vi "MegaAnalysis5.vi"() -> ()   [LabVIEW 2016] (continued)
                    n131 = property on="data column selection" class="Arr (strict)"("Val(Sgnl)"=w337) -> ()  [unwired: 2 in, 2 out]
                  }
                }
              }
              frame #4 {
                n132 = case shown="False" "clear arrays" {
                  tunnel: w339 -> [_ w340]
                  frame False {
                  }
                  frame True {
                    n133 = property on="data column selection" class="Arr (strict)"("Val(Sgnl)"=w340) -> ()  [unwired: 2 in, 2 out]
                    n134 = property on="data column rescale" class="Arr (strict)"("Val(Sgnl)"=w340) -> ()  [unwired: 2 in, 2 out]
                    n135 = property on="data column offset" class="Arr (strict)"("Val(Sgnl)"=w340) -> ()  [unwired: 2 in, 2 out]
                  }
                }
              }
            }
          }
          frame #8 {
            n136 = case shown="True" "?" {
              frame False {
              }
              frame True {
                n137 = Build Array(path "") -> (w360:path[])
                n138 = property on="files to be imported" class="Arr (strict)"("Val(Sgnl)"=w360) -> ()  [unwired: 2 in, 2 out]
              }
            }
            n139 = case shown="False" "divide amplitude rescale amplitude by Sin(2 x angle of B field)" {
              tunnel: w341 -> [_ w358]
              tunnel: w343 -> [_ w359]
              frame False {
              }
              frame True {
                n140 = Unbundle(w359) -> ("data column rescale"=w349:ext[])  [unwired: 4 out]
                n141 = Divide(x=w358, y=180) -> (x/y=w356:ext[])
                n142 = Multiply(x=w356, y=3.141592653589793) -> (x*y=w354:ext[])
                n143 = Multiply(x=2, y=w354) -> (x*y=w352:ext[])
                n144 = Sine(x=w352) -> (sin(x)=w351:ext[])
                n145 = Divide(x=w349, y=w351) -> (x/y=w350:ext[])
                n146 = property on="data column rescale" class="Arr (strict)"("Val(Sgnl)"=w350) -> ()  [unwired: 2 in, 2 out]
              }
            }
            n147 = case shown="False" "increment all angles (theta) by:" {
              tunnel: w341 -> [_ w347]
              frame False {
              }
              frame True {
                n148 = Add(x="?", y=w347) -> (x+y=w346:ext[])
                n149 = property on="angle theta (cos theta renorm.)" class="Arr (strict)"("Val(Sgnl)"=w346) -> ()  [unwired: 2 in, 2 out]
              }
            }
          }
          frame #9 {
            n150 = for {
              tunnel: w374 -> [w379] mode=indexing
              tunnel: [w379] -> w373 mode=indexing
              tunnel: [w381] -> w364 mode=indexing
              tunnel: [w380] -> _ mode=indexing
              n151 = Strip Path(path=w379) -> (stripped path=w380:path, name=w381:string)
            }
            n152 = Build Array(w365, w364) -> (w362:string[][])
            n153 = Transpose 2D Array(2D array=w362) -> (transposed array=→"file list":string[][])
            n154 = case shown="True" w369 {
              tunnel: w378 -> [_ w391]
              tunnel: w377 -> [_ w395]
              tunnel: w376 -> [_ w394]
              tunnel: w375 -> [_ w393]
              tunnel: w373 -> [_ w390]
              tunnel: w372 -> [_ w389]
              tunnel: w371 -> [_ w388]
              tunnel: "file format" -> [_ w387]
              tunnel: w368 -> [_ w384]
              tunnel: w367 -> [_ w383]
              tunnel: w366 -> [_ w382]
              frame False {
              }
              frame True {
                n155 = for {
                  tunnel: w395 -> [w418]
                  tunnel: w391 -> [w417]
                  tunnel: w394 -> [w416]
                  tunnel: w393 -> [w415]
                  tunnel: w387 -> [w414]
                  tunnel: "skip" -> [w403]
                  tunnel: w390 -> [w399] mode=indexing
                  tunnel: w389 -> [w406]
                  tunnel: w388 -> [w405]
                  tunnel: [w404] -> w386 mode=indexing
                  tunnel: [w402] -> w385 mode=indexing
                  tunnel: w384 -> [w401]
                  tunnel: w383 -> [w397]
                  tunnel: w382 -> [w400]
                  i -> [w419]
                  n156 = call "tmdsverify.vi"("file path"=w399) -> ("Boolean"=w398:bool)  [unwired: 10 in]
                  n157 = case shown="True" w398 {
                    tunnel: w414 -> [w423 _]
                    tunnel: [w422 w426] -> w408
                    tunnel: w399 -> [w421 w427]
                    tunnel: w397 -> [w420 _]
                    tunnel: [w420 w425] -> w396
                    frame False {
                      n158 = call-poly <vilib>:"Read From Spreadsheet File.vi"("format (%.3f)"=w423, "file path (dialog if empty)"=w421) -> ("all rows"=w422:dbl[][])  [unwired: 2 in, 7 out]
                    }
                    frame True {
                      n159 = local read "Group name"() -> (w424:string)
                      n160 = call "TDMSextractspreadsheet.vi"("Group name"=w424, "file path"=w427) -> ("dt"=w425:dbl, "data"=w426:dbl[][])  [unwired: 7 in, 1 out]
                    }
                  }
                  n161 = Array Size(array=w408) -> (size(s)=w411:i32[])
                  n162 = Index Array(array=w411, index=0) -> (element=w410:i32)
                  n163 = Index Array(array=w411, index=1) -> (element=w402:i32)
                  n164 = Subtract(x=w410, y=w403) -> (x-y=w404:i32)
                  n165 = Array Subset(array=w408, index (row)=w403, length (row)=w404, index (col)=0, length (col)=w402) -> (w407:dbl[][])
                  n166 = stacked-sequence {
                    seq-local: [w434 _ _ _ _ _ _ _] -> [_ _ w531 w612 w680 _ _ _]
                    tunnel: w407 -> [w442 w483 w535 w613 w681 _ w756 _]
                    tunnel: w419 -> [w430 w474 w519 w599 w663 w731 w748 w758]
                    tunnel: w418 -> [w429 w473 w518 w598 w662 w730 w747 w759]
                    tunnel: w417 -> [w441 w484 w536 w614 w682 _ _ _]
                    tunnel: w416 -> [w440 w489 w539 w617 w685 _ _ _]
                    tunnel: w415 -> [w439 w490 w540 w618 w686 _ _ _]
                    tunnel: w406 -> [_ _ w530 w609 w679 _ _ _]
                    tunnel: w405 -> [_ _ w527 w602 w672 _ _ _]
                    tunnel: w401 -> [w432 w476 w521 w593 w661 w729 w751 w760]
                    tunnel: w396 -> [w428 _ _ _ _ _ _ _]
                    tunnel: w400 -> [_ _ w514 _ _ _ _ _]
                    frame #0 {
                      # "time"
                      n167 = Unbundle(w440) -> ("time column selection"=w438:u16[])  [unwired: 4 out]
                      n168 = Unbundle(w439) -> ("time column rescale"=w437:ext[])  [unwired: 4 out]
                      n169 = case shown="1" w441 {
                        tunnel: [w447 w450] -> w435
                        tunnel: [w446 w449] -> w436
                        tunnel: w438 -> [w445 w453]
                        tunnel: w437 -> [w444 w452]
                        tunnel: w430 -> [_ w451]
                        frame 0, Default {
                          w448 = 0
                          n170 = Index Array(array=w444, index=w448) -> (element=w446:ext)
                          n171 = Index Array(array=w445, index=w448) -> (element=w447:u16)
                        }
                        frame 1 {
                          n172 = Index Array(array=w453, index=w451) -> (element=w450:u16)
                          n173 = Index Array(array=w452, index=w451) -> (element=w449:ext)
                        }
                      }
                      n174 = case shown="2" "option" {
                        tunnel: [dbl[] [] ("Array 3") w457 w468] -> w433
                        tunnel: w442 -> [_ w465 w470]
                        tunnel: w436 -> [_ w463 _]
                        tunnel: w435 -> [_ w462 _]
                        tunnel: [w454 w456 w466] -> w434
                        tunnel: w428 -> [w454 _ w466]
                        frame 0, Default {
                        }
                        frame 1 {
                          n175 = Index Array(array=w465, index (col)=w462) -> (element=w464:dbl[])  [unwired: 1 in]
                          n176 = Multiply(x=w464, y=w463) -> (x*y=w457:ext[])
                          n177 = Index Array(array=w457, index=0) -> (element=w459:ext)
                          n178 = Index Array(array=w457, index=1) -> (element=w458:ext)
                          n179 = Subtract(x=w458, y=w459) -> (x-y=w456:ext)
                        }
                        frame 2 {
                          n180 = Index Array(array=w470, index (col)=0) -> (element=w469:dbl[])  [unwired: 1 in]
                          n181 = for {
                            tunnel: [w472] -> w467 mode=indexing
                            tunnel: w469 -> [_] mode=indexing
                            i -> [w472]
                          }
                          n182 = Multiply(x=w467, y=w466) -> (x*y=w468:dbl[])
                        }
                      }
                      n183 = property on="time interval  (for series)" class="DigNum (strict)"("Val(Sgnl)"=w428) -> ()  [unwired: 2 in, 2 out]
                      n184 = call "writebinary.vi"(7:w432, "base path"=w429, "file index"=w430, "data column"="time", "data"=w433) -> ()  [unwired: 7 out]
                    }
                    frame #1 {
                      w475 = "bdot"
                      (unwired) 3
                      # "bdot"
                      n185 = Unbundle(w489) -> ("dB/dt column selection"=w488:u16[])  [unwired: 4 out]
                      n186 = Unbundle(w490) -> ("dB/dt column rescale"=w487:ext[])  [unwired: 4 out]
                      n187 = case shown="1" w484 {
                        tunnel: [w495 w501] -> w486
                        tunnel: [w494 w500] -> w485
                        tunnel: w488 -> [w493 w499]
                        tunnel: w487 -> [w492 w498]
                        tunnel: w474 -> [_ w497]
                        frame 0, Default {
                          w496 = 0
                          n188 = Index Array(array=w492, index=w496) -> (element=w494:ext)
                          n189 = Index Array(array=w493, index=w496) -> (element=w495:u16)
                        }
                        frame 1 {
                          n190 = Index Array(array=w499, index=w497) -> (element=w501:u16)
                          n191 = Index Array(array=w498, index=w497) -> (element=w500:ext)
                        }
                      }
                      n192 = case shown="0, Default" "option" {
                        tunnel: [dbl[] [] ("Array 5") w505] -> w477
                        tunnel: w483 -> [_ w507]
                        tunnel: w486 -> [_ w504]
                        tunnel: w485 -> [_ w503]
                        frame 0, Default {
                        }
                        frame 1 {
                          n193 = Index Array(array=w507, index (col)=w504) -> (element=w506:dbl[])  [unwired: 1 in]
                          n194 = Multiply(x=w506, y=w503) -> (x*y=w505:ext[])
                        }
                      }
                      n195 = Number To Decimal String(number=w474, width (-)=2) -> (decimal integer string=w481:string)
                      n196 = call "writebinary.vi"(7:w476, "base path"=w473, "file index"=w474, "data column"=w475, "data"=w477) -> ()  [unwired: 7 out]
                      n197 = Search and Replace String(input string=w481, search string=" ", replace string="0") -> (result string=w478:string)  [unwired: 2 in, 6 out]
                      n198 = Concatenate Strings(w478, w475) -> ()  [unwired: 1 out]
                    }
                    frame #2 {
                      # "Bcol"
                      n199 = Unbundle(w539) -> ("B column selection"=w533:u16[])  [unwired: 4 out]
                      n200 = Unbundle(w540) -> ("B column rescale"=w532:ext[])  [unwired: 4 out]
                      n201 = Unbundle(w530) -> ("B column offset"=w529:ext[])  [unwired: 2 out]
                      n202 = case shown="1" w536 {
                        tunnel: [w562 w571] -> w538
                        tunnel: [w561 w570] -> w537
                        tunnel: w533 -> [w560 w569]
                        tunnel: w532 -> [w559 w568]
                        tunnel: w519 -> [_ w564]
                        tunnel: w529 -> [w558 w567]
                        tunnel: [w557 w566] -> w523
                        tunnel: w514 -> [w556 w563]
                        tunnel: [w555 w565] -> w512
                        frame 0, Default {
                          w554 = 0
                          n203 = Index Array(array=w558, index=w554) -> (element=w557:ext)
                          n204 = Index Array(array=w556, index=w554) -> (element=w555:ext)
                          n205 = Index Array(array=w559, index=w554) -> (element=w561:ext)
                          n206 = Index Array(array=w560, index=w554) -> (element=w562:u16)
                        }
                        frame 1 {
                          n207 = Index Array(array=w569, index=w564) -> (element=w571:u16)
                          n208 = Index Array(array=w567, index=w564) -> (element=w566:ext)
                          n209 = Index Array(array=w568, index=w564) -> (element=w570:ext)
                          n210 = Index Array(array=w563, index=w564) -> (element=w565:ext)
                        }
                      }
                      n211 = Unbundle(w527) -> ("pretrigger time for integration"=w526:dbl)  [unwired: 2 out]
                      n212 = case shown="0, Default" "option" {
                        tunnel: [dbl[] [] ("Array 6") w575 w582 w592] -> w525
                        tunnel: w535 -> [_ w577 w583 _]
                        tunnel: w538 -> [_ w574 w581 _]
                        tunnel: w537 -> [_ w573 w580 _]
                        tunnel: w531 -> [_ _ _ w591]
                        tunnel: w526 -> [_ _ _ w589]
                        tunnel: w521 -> [_ _ _ w588]
                        tunnel: w519 -> [_ _ _ w586]
                        tunnel: w518 -> [_ _ _ w585]
                        frame 0, Default {
                        }
                        frame 1 {
                          n213 = Index Array(array=w577, index (col)=w574) -> (element=w576:dbl[])  [unwired: 1 in]
                          n214 = Multiply(x=w576, y=w573) -> (x*y=w575:ext[])
                        }
                        frame 2 {
                          n215 = Index Array(array=w583, index (col)=w581) -> (element=w579:dbl[])  [unwired: 1 in]
                          n216 = Reciprocal(x=w579) -> (1/x=w578:dbl[])
                          n217 = Multiply(x=w578, y=w580) -> (x*y=w582:ext[])
                        }
                        frame 3 {
                          n218 = call "readbinary.vi"(7:w588, "base path"=w585, "file index"=w586, "data column"="bdot") -> ("data"=w584:ext[])  [unwired: 7 out]
                          n219 = call "integrator2.vi"("reverse intergral"="?", "pretrigger t"=w589, "dt"=w591, "data"=w584) -> ("integrated data"=w592:dbl[])  [unwired: 2 in]
                        }
                      }
                      n220 = Divide(x=w512, y=180) -> (x/y=w516:ext)
                      n221 = Multiply(x=w516, y=3.141592653589793) -> (x*y=w513:ext)
                      n222 = Cosine(x=w513) -> (cos(x)=w511:ext)
                      n223 = case shown="True" "?" {
                        tunnel: w525 -> [w544 w546]
                        tunnel: [w544 w545] -> w524
                        frame False {
                        }
                        frame True {
                          n224 = Absolute Value(x=w546) -> (abs(x)=w550:ext[])
                          n225 = Array Max & Min(array=w550) -> (max index (indices)=w549:i32)  [unwired: 3 out]
                          n226 = Index Array(array=w546, index=w549) -> (element=w548:ext)
                          n227 = Sign(1:w548) -> (0:w547:ext)
                          n228 = Multiply(x=w546, y=w547) -> (x*y=w545:ext[])
                        }
                      }
                      n229 = case shown="False" "?" {
                        tunnel: w523 -> [w542 w543]
                        tunnel: [w541 w543] -> _
                        frame False {
                          n230 = To Double Precision Float(number=w542) -> (double precision float=w541:dbl)
                        }
                        frame True {
                        }
                      }
                      n231 = case shown="False" "?" {
                        tunnel: w524 -> [w551 w553]
                        tunnel: [w551 w552] -> w510
                        frame False {
                        }
                        frame True {
                          n232 = call "forceBendtozero2.vi"("data"=w553) -> ("forced data"=w552:dbl[])
                        }
                      }
                      n233 = Add(x=w523, y=w510) -> (x+y=w509:ext[])
                      n234 = Multiply(x=w509, y=w511) -> (x*y=w508:ext[])
                      n235 = call "writebinary.vi"(7:w521, "base path"=w518, "file index"=w519, "data column"="bcol", "data"=w508) -> ()  [unwired: 7 out]
                    }
                    frame #3 {
                      # "data1"
                      n236 = Unbundle(w617) -> ("data column selection"=w610:u16[])  [unwired: 4 out]
                      n237 = Unbundle(w618) -> ("data column rescale"=w611:ext[])  [unwired: 4 out]
                      n238 = Unbundle(w609) -> ("data column offset"=w608:ext[])  [unwired: 2 out]
                      n239 = case shown="0, Default" w614 {
                        tunnel: [w632 w639] -> w616
                        tunnel: [w631 w638] -> w615
                        tunnel: w610 -> [w630 w637]
                        tunnel: w611 -> [w629 w636]
                        tunnel: w599 -> [_ w634]
                        tunnel: w608 -> [w628 w635]
                        tunnel: [w626 w633] -> w607
                        frame 0, Default {
                          w627 = 0
                          n240 = Index Array(array=w628, index=w627) -> (element=w626:ext)
                          n241 = Index Array(array=w629, index=w627) -> (element=w631:ext)
                          n242 = Index Array(array=w630, index=w627) -> (element=w632:u16)
                        }
                        frame 1 {
                          n243 = Index Array(array=w635, index=w634) -> (element=w633:ext)
                          n244 = Index Array(array=w637, index=w634) -> (element=w639:u16)
                          n245 = Index Array(array=w636, index=w634) -> (element=w638:ext)
                        }
                      }
                      n246 = Unbundle(w602) -> ("pretrigger time for integration"=w601:dbl)  [unwired: 2 out]
                      n247 = case shown="0, Default" "option" {
                        tunnel: [dbl[] [] ("Array 7") w643 w650 w660] -> w604
                        tunnel: w613 -> [_ w645 w651 w657]
                        tunnel: w616 -> [_ w642 w649 w656]
                        tunnel: w615 -> [_ w641 w648 w652]
                        tunnel: w612 -> [_ _ _ w659]
                        tunnel: w601 -> [_ _ _ w654]
                        frame 0, Default {
                        }
                        frame 1 {
                          n248 = Index Array(array=w645, index (col)=w642) -> (element=w644:dbl[])  [unwired: 1 in]
                          n249 = Multiply(x=w644, y=w641) -> (x*y=w643:ext[])
                        }
                        frame 2 {
                          n250 = Index Array(array=w651, index (col)=w649) -> (element=w647:dbl[])  [unwired: 1 in]
                          n251 = Reciprocal(x=w647) -> (1/x=w646:dbl[])
                          n252 = Multiply(x=w646, y=w648) -> (x*y=w650:ext[])
                        }
                        frame 3 {
                          n253 = Index Array(array=w657, index (col)=w656) -> (element=w655:dbl[])  [unwired: 1 in]
                          n254 = Multiply(x=w652, y=w655) -> (x*y=w653:ext[])
                          n255 = call "integrator2.vi"("reverse intergral"="?", "pretrigger t"=w654, "dt"=w659, "data"=w653) -> ("integrated data"=w660:dbl[])  [unwired: 2 in]
                        }
                      }
                      n256 = case shown="False" "?" {
                        tunnel: w604 -> [w623 w625]
                        tunnel: [w623 w624] -> w603
                        frame False {
                        }
                        frame True {
                          n257 = call "forceBendtozero2.vi"("data"=w625) -> ("forced data"=w624:dbl[])
                        }
                      }
                      n258 = Add(x=w607, y=w603) -> (x+y=w596:ext[])
                      n259 = case shown="True" "?" {
                        tunnel: w596 -> [w619 w622]
                        tunnel: "?" -> [_ w621]
                        tunnel: [w619 w620] -> w594
                        frame False {
                        }
                        frame True {
                          n260 = Rotate 1D Array(1:w622, 2:w621) -> (0:w620:ext[])
                        }
                      }
                      n261 = call "writebinary.vi"(7:w593, "base path"=w598, "file index"=w599, "data column"="dat1", "data"=w594) -> ()  [unwired: 7 out]
                    }
                    frame #4 {
                      # "data2"
                      n262 = Unbundle(w685) -> ("data column selection"=w669:u16[])  [unwired: 4 out]
                      n263 = Unbundle(w686) -> ("data column rescale"=w670:ext[])  [unwired: 4 out]
                      n264 = Unbundle(w679) -> ("data column offset"=w678:ext[])  [unwired: 2 out]
                      n265 = case shown="0, Default" w682 {
                        tunnel: [w700 w707] -> w684
                        tunnel: [w699 w706] -> w683
                        tunnel: w669 -> [w698 w705]
                        tunnel: w670 -> [w697 w704]
                        tunnel: w663 -> [_ w702]
                        tunnel: w678 -> [w696 w703]
                        tunnel: [w694 w701] -> w677
                        frame 0, Default {
                          w695 = 0
                          n266 = Index Array(array=w696, index=w695) -> (element=w694:ext)
                          n267 = Index Array(array=w697, index=w695) -> (element=w699:ext)
                          n268 = Index Array(array=w698, index=w695) -> (element=w700:u16)
                        }
                        frame 1 {
                          n269 = Index Array(array=w703, index=w702) -> (element=w701:ext)
                          n270 = Index Array(array=w705, index=w702) -> (element=w707:u16)
                          n271 = Index Array(array=w704, index=w702) -> (element=w706:ext)
                        }
                      }
                      n272 = Unbundle(w672) -> ("pretrigger time for integration"=w671:dbl)  [unwired: 2 out]
                      n273 = case shown="0, Default" "option" {
                        tunnel: [dbl[] [] ("Array 8") w711 w718 w728] -> w673
                        tunnel: w681 -> [_ w713 w719 w726]
                        tunnel: w684 -> [_ w710 w717 w725]
                        tunnel: w683 -> [_ w709 w716 w720]
                        tunnel: w680 -> [_ _ _ w727]
                        tunnel: w671 -> [_ _ _ w722]
                        frame 0, Default {
                        }
                        frame 1 {
                          n274 = Index Array(array=w713, index (col)=w710) -> (element=w712:dbl[])  [unwired: 1 in]
                          n275 = Multiply(x=w712, y=w709) -> (x*y=w711:ext[])
                        }
                        frame 2 {
                          n276 = Index Array(array=w719, index (col)=w717) -> (element=w715:dbl[])  [unwired: 1 in]
                          n277 = Reciprocal(x=w715) -> (1/x=w714:dbl[])
                          n278 = Multiply(x=w714, y=w716) -> (x*y=w718:ext[])
                        }
                        frame 3 {
                          n279 = Index Array(array=w726, index (col)=w725) -> (element=w724:dbl[])  [unwired: 1 in]
                          n280 = Multiply(x=w720, y=w724) -> (x*y=w721:ext[])
                          n281 = call "integrator2.vi"("reverse intergral"="?", "pretrigger t"=w722, "dt"=w727, "data"=w721) -> ("integrated data"=w728:dbl[])  [unwired: 2 in]
                        }
                      }
                      n282 = case shown="False" "?" {
                        tunnel: w673 -> [w691 w693]
                        tunnel: [w691 w692] -> w674
                        frame False {
                        }
                        frame True {
                          n283 = call "forceBendtozero2.vi"("data"=w693) -> ("forced data"=w692:dbl[])
                        }
                      }
                      n284 = Add(x=w677, y=w674) -> (x+y=w668:ext[])
                      n285 = case shown="True" "?" {
                        tunnel: w668 -> [w687 w690]
                        tunnel: "?" -> [_ w689]
                        tunnel: [w687 w688] -> w665
                        frame False {
                        }
                        frame True {
                          n286 = Rotate 1D Array(1:w690, 2:w689) -> (0:w688:ext[])
                        }
                      }
                      n287 = call "writebinary.vi"(7:w661, "base path"=w662, "file index"=w663, "data column"="dat2", "data"=w665) -> ()  [unwired: 7 out]
                    }
                    frame #5 {
                      n288 = case shown="True" "?" {
                        tunnel: w731 -> [_ w735]
                        tunnel: w730 -> [_ w733]
                        tunnel: w729 -> [_ w734]
                        frame False {
                        }
                        frame True {
                          w742 = -1
                          n289 = call "readbinary.vi"(7:w734, "base path"=w733, "file index"=w735, "data column"="time") -> ("data"=w740:ext[])  [unwired: 7 out]
                          n290 = call "readbinary.vi"(7:w734, "base path"=w733, "file index"=w735, "data column"="bcol") -> ("data"=w743:ext[])  [unwired: 7 out]
                          n291 = Rotate 1D Array(1:w740, 2:w742) -> (0:w741:ext[])
                          n292 = Rotate 1D Array(1:w743, 2:w742) -> (0:w744:ext[])
                          n293 = Subtract(x=w740, y=w741) -> (x-y=w738:ext[])
                          n294 = Subtract(x=w743, y=w744) -> (x-y=w739:ext[])
                          n295 = Divide(x=w739, y=w738) -> (x/y=w737:ext[])
                          n296 = call "writebinary.vi"(7:w734, "base path"=w733, "file index"=w735, "data column"="bdot", "data"=w737) -> ()  [unwired: 7 out]
                        }
                      }
                    }
                    frame #6 {
                      n297 = Array Size(array=w756) -> (size(s)=w755:i32[])
                      n298 = Index Array(array=w755, index=0) -> (element=w753:i32)
                      n299 = for {
                        N: w753 -> [_]
                        tunnel: [w757] -> w752 mode=indexing
                        i -> [w757]
                      }
                      n300 = To Extended Precision Float(1:w752) -> (0:w750:ext[])
                      n301 = call "writebinary.vi"(7:w751, "base path"=w747, "file index"=w748, "data column"="indx", "data"=w750) -> ()  [unwired: 7 out]
                    }
                    frame #7 {
                      n302 = case shown="True" "?" {
                        tunnel: w760 -> [_ w764]
                        tunnel: w759 -> [_ w765]
                        tunnel: w758 -> [_ w766]
                        frame False {
                        }
                        frame True {
                          w784 = dbl[] [] ("Array 25")
                          n303 = call "readbinary.vi"(7:w764, "base path"=w765, "file index"=w766, "data column"="dat2") -> ("data"=w783:ext[])  [unwired: 7 out]
                          n304 = call "readbinary.vi"(7:w764, "base path"=w765, "file index"=w766, "data column"="indx") -> ("data"=w763:ext[])  [unwired: 7 out]
                          n305 = Array Size(array=w763) -> (size(s)=w762:i32)
                          n306 = call "readbinary.vi"(7:w764, "base path"=w765, "file index"=w766, "data column"="dat1") -> ("data"=w782:ext[])  [unwired: 7 out]
                          n307 = call "readbinary.vi"(7:w764, "base path"=w765, "file index"=w766, "data column"="time") -> ("data"=w780:ext[])  [unwired: 7 out]
                          n308 = call "readbinary.vi"(7:w764, "base path"=w765, "file index"=w766, "data column"="bdot") -> ("data"=w781:ext[])  [unwired: 7 out]
                          n309 = call "readbinary.vi"(7:w764, "base path"=w765, "file index"=w766, "data column"="bcol") -> ("data"=w779:ext[])  [unwired: 7 out]
                          n310 = for {
                            N: w762 -> [_]
                            shift-right: [w807] -> w778
                            shift-left: w784 -> [w808]
                            shift-right: [w805] -> w777
                            shift-left: w784 -> [w806]
                            shift-right: [w804] -> w776
                            shift-left: w784 -> [w803]
                            shift-right: [w802] -> w775
                            shift-left: w784 -> [w801]
                            shift-right: [w800] -> w774
                            shift-left: w784 -> [w799]
                            shift-right: [w798] -> w773
                            shift-left: w784 -> [w797]
                            tunnel: w763 -> [w816]
                            tunnel: w783 -> [w815]
                            tunnel: w782 -> [w814]
                            tunnel: w781 -> [w813]
                            tunnel: w780 -> [w812]
                            tunnel: w779 -> [w811]
                            i -> [w810]
                            n311 = Index Array(array=w812, index=w810) -> (element=w795:ext)
                            n312 = Index Array(array=w816, index=w810) -> (element=w791:ext)
                            n313 = Index Array(array=w815, index=w810) -> (element=w792:ext)
                            n314 = Index Array(array=w811, index=w810) -> (element=w796:ext)
                            n315 = Equal To 0?(x=w796) -> (x = 0?=w809:bool)
                            n316 = Index Array(array=w814, index=w810) -> (element=w793:ext)
                            n317 = Index Array(array=w813, index=w810) -> (element=w794:ext)
                            n318 = case shown="False" w809 {
                              tunnel: w808 -> [w834 w840]
                              tunnel: [w822 w840] -> w807
                              tunnel: w806 -> [w833 w839]
                              tunnel: [w821 w839] -> w805
                              tunnel: [w818 w838] -> w804
                              tunnel: w803 -> [w832 w838]
                              tunnel: [w819 w837] -> w802
                              tunnel: w801 -> [w831 w837]
                              tunnel: [w820 w836] -> w800
                              tunnel: w799 -> [w830 w836]
                              tunnel: [w817 w835] -> w798
                              tunnel: w797 -> [w829 w835]
                              tunnel: w796 -> [w828 _]
                              tunnel: w795 -> [w827 _]
                              tunnel: w794 -> [w826 _]
                              tunnel: w793 -> [w825 _]
                              tunnel: w792 -> [w824 _]
                              tunnel: w791 -> [w823 _]
                              frame False {
                                n319 = Build Array (concatenate)(w829, w823) -> (w817:ext[])
                                n320 = Build Array (concatenate)(w830, w824) -> (w820:ext[])
                                n321 = Build Array (concatenate)(w833, w827) -> (w821:ext[])
                                n322 = Build Array (concatenate)(w831, w825) -> (w819:ext[])
                                n323 = Build Array (concatenate)(w834, w828) -> (w822:ext[])
                                n324 = Build Array (concatenate)(w832, w826) -> (w818:ext[])
                              }
                              frame True {
                              }
                            }
                          }
                          n325 = call "writebinary.vi"(7:w764, "base path"=w765, "file index"=w766, "data column"="dat2", "data"=w774) -> ()  [unwired: 7 out]
                          n326 = call "writebinary.vi"(7:w764, "base path"=w765, "file index"=w766, "data column"="time", "data"=w777) -> ()  [unwired: 7 out]
                          n327 = call "writebinary.vi"(7:w764, "base path"=w765, "file index"=w766, "data column"="indx", "data"=w773) -> ()  [unwired: 7 out]
                          n328 = call "writebinary.vi"(7:w764, "base path"=w765, "file index"=w766, "data column"="dat1", "data"=w775) -> ()  [unwired: 7 out]
                          n329 = call "writebinary.vi"(7:w764, "base path"=w765, "file index"=w766, "data column"="bcol", "data"=w778) -> ()  [unwired: 7 out]
                          n330 = call "writebinary.vi"(7:w764, "base path"=w765, "file index"=w766, "data column"="bdot", "data"=w776) -> ()  [unwired: 7 out]
                        }
                      }
                    }
                  }
                }
                "# columns" <- w385
                "# rows" <- w386
              }
            }
          }
          frame #10 {
            n331 = case shown="True" "read angle from data 2 index:" {
              tunnel: w844 -> [_ w848]
              tunnel: w843 -> [_ w849]
              tunnel: w842 -> [_ w847]
              frame False {
              }
              frame True {
                n332 = for {
                  tunnel: w849 -> [w856]
                  tunnel: w848 -> [_] mode=indexing
                  tunnel: w847 -> [w854]
                  tunnel: "?" -> [w852]
                  tunnel: [w850] -> w845 mode=indexing
                  i -> [w853]
                  n333 = call "readbinary.vi"(7:w856, "base path"=w854, "file index"=w853, "data column"="dat2") -> ("data"=w851:ext[])  [unwired: 7 out]
                  n334 = Index Array(array=w851, index=w852) -> (element=w850:ext)
                }
                n335 = property on="angle theta (cos theta renorm.)" class="Arr (strict)"("Val(Sgnl)"=w845) -> ()  [unwired: 2 in, 2 out]
              }
            }
          }
          frame #11 {
            n336 = case shown="True" "make all files have same settings as file 0" {
              tunnel: w857 -> [_ w859]
              frame False {
              }
              frame True {
                n337 = stacked-sequence {
                  tunnel: w859 -> [w860 w871 w891 w906 w925]
                  frame #0 {
                    n338 = property on="time column selection" class="Arr (strict)"() -> ("Value"=w864:u16[])  [unwired: 2 in, 2 out]
                    n339 = property on="time column rescale" class="Arr (strict)"() -> ("Value"=w863:ext[])  [unwired: 2 in, 2 out]
                    n340 = Index Array(array=w864, index=0) -> (element=w866:u16)
                    n341 = Index Array(array=w863, index=0) -> (element=w865:ext)
                    n342 = for {
                      tunnel: w866 -> [w870]
                      tunnel: w865 -> [w869]
                      tunnel: [w870] -> w862 mode=indexing
                      tunnel: [w869] -> w861 mode=indexing
                      tunnel: w860 -> [_] mode=indexing
                    }
                    n343 = property on="time column selection" class="Arr (strict)"("Val(Sgnl)"=w862) -> ()  [unwired: 2 in, 2 out]
                    n344 = property on="time column rescale" class="Arr (strict)"("Val(Sgnl)"=w861) -> ()  [unwired: 2 in, 2 out]
                  }
                  frame #1 {
                    n345 = property on="dB/dt column rescale" class="Arr (strict)"() -> ("Value"=w874:ext[])  [unwired: 2 in, 2 out]
                    n346 = property on="dB/dt column selection" class="Arr (strict)"() -> ("Value"=w875:u16[])  [unwired: 2 in, 2 out]
                    n347 = Index Array(array=w875, index=0) -> (element=w877:u16)
                    n348 = Index Array(array=w874, index=0) -> (element=w876:ext)
                    n349 = for {
                      tunnel: w877 -> [w881]
                      tunnel: w876 -> [w880]
                      tunnel: [w881] -> w873 mode=indexing
                      tunnel: [w880] -> w872 mode=indexing
                      tunnel: w871 -> [_] mode=indexing
                    }
                    n350 = property on="dB/dt column rescale" class="Arr (strict)"("Val(Sgnl)"=w872) -> ()  [unwired: 2 in, 2 out]
                    n351 = property on="dB/dt column selection" class="Arr (strict)"("Val(Sgnl)"=w873) -> ()  [unwired: 2 in, 2 out]
                  }
                  frame #2 {
                    n352 = local read "B column selection"() -> (w882:u16[])
                    n353 = property on="B column rescale" class="Arr (strict)"() -> ("Value"=w894:ext[])  [unwired: 2 in, 2 out]
                    n354 = property on="angle theta (cos theta renorm.)" class="Arr (strict)"() -> ("Value"=w893:ext[])  [unwired: 2 in, 2 out]
                    n355 = property on="B column offset" class="Arr (strict)"() -> ("Value"=w892:ext[])  [unwired: 2 in, 2 out]
                    n356 = Index Array(array=w882, index=0) -> (element=w890:u16)
                    n357 = Index Array(array=w892, index=0) -> (element=w887:ext)
                    n358 = Index Array(array=w894, index=0) -> (element=w889:ext)
                    n359 = Index Array(array=w893, index=0) -> (element=w888:ext)
                    n360 = for {
                      tunnel: w891 -> [_] mode=indexing
                      tunnel: w890 -> [w902]
                      tunnel: w889 -> [w901]
                      tunnel: w888 -> [w900]
                      tunnel: w887 -> [w899]
                      tunnel: [w902] -> w883 mode=indexing
                      tunnel: [w901] -> w886 mode=indexing
                      tunnel: [w900] -> w885 mode=indexing
                      tunnel: [w899] -> w884 mode=indexing
                    }
                    n361 = property on="B column offset" class="Arr (strict)"("Val(Sgnl)"=w884) -> ()  [unwired: 2 in, 2 out]
                    n362 = property on="angle theta (cos theta renorm.)" class="Arr (strict)"("Val(Sgnl)"=w885) -> ()  [unwired: 2 in, 2 out]
                    n363 = property on="B column rescale" class="Arr (strict)"("Val(Sgnl)"=w886) -> ()  [unwired: 2 in, 2 out]
                    n364 = local write "B column selection"(w883) -> ()
                  }
                  frame #3 {
                    n365 = property on="data column rescale" class="Arr (strict)"() -> ("Value"=w908:ext[])  [unwired: 2 in, 2 out]
                    n366 = property on="data column selection" class="Arr (strict)"() -> ("Value"=w909:u16[])  [unwired: 2 in, 2 out]
                    n367 = property on="data column offset" class="Arr (strict)"() -> ("Value"=w907:ext[])  [unwired: 2 in, 2 out]
                    n368 = Index Array(array=w909, index=0) -> (element=w912:u16)
                    n369 = Index Array(array=w908, index=0) -> (element=w911:ext)
                    n370 = Index Array(array=w907, index=0) -> (element=w910:ext)
                    n371 = for {
                      tunnel: w912 -> [w918]
                      tunnel: w911 -> [w917]
                      tunnel: w910 -> [w916]
                      tunnel: [w918] -> w905 mode=indexing
                      tunnel: [w917] -> w904 mode=indexing
                      tunnel: [w916] -> w903 mode=indexing
                      tunnel: w906 -> [_] mode=indexing
                    }
                    n372 = property on="data column rescale" class="Arr (strict)"("Val(Sgnl)"=w904) -> ()  [unwired: 2 in, 2 out]
                    n373 = property on="data column offset" class="Arr (strict)"("Val(Sgnl)"=w903) -> ()  [unwired: 2 in, 2 out]
                    n374 = property on="data column selection" class="Arr (strict)"("Val(Sgnl)"=w905) -> ()  [unwired: 2 in, 2 out]
                  }
                  frame #4 {
                    n375 = property on="data column rescale" class="Arr (strict)"() -> ("Value"=w923:ext[])  [unwired: 2 in, 2 out]
                    n376 = property on="data column selection" class="Arr (strict)"() -> ("Value"=w924:u16[])  [unwired: 2 in, 2 out]
                    n377 = property on="data column offset" class="Arr (strict)"() -> ("Value"=w922:ext[])  [unwired: 2 in, 2 out]
                    n378 = Index Array(array=w924, index=0) -> (element=w928:u16)
                    n379 = Index Array(array=w923, index=0) -> (element=w927:ext)
                    n380 = Index Array(array=w922, index=0) -> (element=w926:ext)
                    n381 = for {
                      tunnel: w928 -> [w934]
                      tunnel: w927 -> [w933]
                      tunnel: w926 -> [w932]
                      tunnel: [w934] -> w921 mode=indexing
                      tunnel: [w933] -> w920 mode=indexing
                      tunnel: [w932] -> w919 mode=indexing
                      tunnel: w925 -> [_] mode=indexing
                    }
                    n382 = property on="data column rescale" class="Arr (strict)"("Val(Sgnl)"=w920) -> ()  [unwired: 2 in, 2 out]
                    n383 = property on="data column selection" class="Arr (strict)"("Val(Sgnl)"=w921) -> ()  [unwired: 2 in, 2 out]
                    n384 = property on="data column offset" class="Arr (strict)"("Val(Sgnl)"=w919) -> ()  [unwired: 2 in, 2 out]
                  }
                }
              }
            }
          }
          frame #12 {
            n385 = case shown="0, Default" "sampling frequency option" {
              tunnel: w940 -> [w944 w957]
              tunnel: w939 -> [w943 _]
              tunnel: [w942 w955] -> w938
              tunnel: w937 -> [w941 _]
              tunnel: w935 -> [_ w956]
              frame 0, Default {
                n386 = for {
                  tunnel: w944 -> [_] mode=indexing
                  tunnel: w943 -> [w952]
                  tunnel: [w946] -> w942 mode=indexing
                  tunnel: w941 -> [w945]
                  i -> [w953]
                  n387 = call "readbinary.vi"(7:w945, "base path"=w952, "file index"=w953, "data column"="time") -> ("data"=w947:ext[])  [unwired: 7 out]
                  n388 = Index Array(array=w947, index=1) -> (element=w950:ext)
                  n389 = Index Array(array=w947, index=0) -> (element=w951:ext)
                  n390 = Subtract(x=w950, y=w951) -> (x-y=w946:ext)
                }
              }
              frame 1 {
                n391 = for {
                  tunnel: w957 -> [_] mode=indexing
                  tunnel: w956 -> [w958]
                  tunnel: [w958] -> w955 mode=indexing
                }
              }
            }
          }
          frame #13 {
            n392 = And(x="?", y=w960) -> (x .and. y?=w961:bool)
            n393 = case shown="True" w961 {
              tunnel: w965 -> [_ w969]
              tunnel: w964 -> [_ w968]
              tunnel: w963 -> [_ w967]
              tunnel: w959 -> [_ w966]
              frame False {
              }
              frame True {
                n394 = for {
                  tunnel: w969 -> [_] mode=indexing
                  tunnel: w968 -> [w973]
                  tunnel: w967 -> [w972]
                  tunnel: w966 -> [w970]
                  i -> [w971]
                  n395 = for {
                    tunnel: w973 -> [w977] mode=indexing
                    tunnel: w972 -> [w976]
                    tunnel: w971 -> [w975]
                    tunnel: w970 -> [w974]
                    n396 = call "readbinary.vi"(7:w974, "base path"=w976, "file index"=w975, "data column"=w977) -> ("data"=w981:ext[])  [unwired: 7 out]
                    n397 = Subtract(x="upper cutoff", y="lower cutoff") -> (x-y=w982:u64)
                    n398 = Increment(x=w982) -> (x+1=w979:u64)
                    n399 = Array Subset(array=w981, index="lower cutoff", length=w979) -> (w978:ext[])
                    n400 = call "writebinary.vi"(7:w974, "base path"=w976, "file index"=w975, "data column"=w977, "data"=w978) -> ()  [unwired: 7 out]
                  }
                }
              }
            }
          }
          frame #14 {
            n401 = And(x="?", y=w986) -> (x .and. y?=w985:bool)
            n402 = case shown="False" w985 {
              tunnel: w990 -> [_ w994]
              tunnel: w989 -> [_ w993]
              tunnel: w988 -> [_ w992]
              tunnel: w984 -> [_ w991]
              frame False {
              }
              frame True {
                n403 = for {
                  tunnel: w994 -> [w997]
                  tunnel: w992 -> [w996]
                  tunnel: w993 -> [_] mode=indexing
                  tunnel: w991 -> [w995]
                  i -> [w998]
                  n404 = stacked-sequence {
                    seq-local: [w1006 _] -> [_ w1014]
                    seq-local: [w1002 _] -> [_ w1013]
                    tunnel: w998 -> [w1010 w1016]
                    tunnel: w997 -> [w1009 w1015]
                    tunnel: w996 -> [_ w1017]
                    tunnel: w995 -> [w999 w1012]
                    frame #0 {
                      n405 = call "readbinary.vi"(7:w999, "base path"=w1009, "file index"=w1010, "data column"="time") -> ("data"=w1003:ext[])  [unwired: 7 out]
                      n406 = Subtract(x=w1003, y="lower cutoff") -> (x-y=w1008:ext[])
                      n407 = Subtract(x=w1003, y="upper cutoff") -> (x-y=w1005:ext[])
                      n408 = Absolute Value(x=w1008) -> (abs(x)=w1007:ext[])
                      n409 = Absolute Value(x=w1005) -> (abs(x)=w1004:ext[])
                      n410 = Array Max & Min(array=w1007) -> (min index (indices)=w1006:i32)  [unwired: 3 out]
                      n411 = Array Max & Min(array=w1004) -> (min index (indices)=w1002:i32)  [unwired: 3 out]
                    }
                    frame #1 {
                      n412 = for {
                        tunnel: w1017 -> [w1023] mode=indexing
                        tunnel: w1016 -> [w1022]
                        tunnel: w1015 -> [w1021]
                        tunnel: w1014 -> [w1019]
                        tunnel: w1013 -> [w1020]
                        tunnel: w1012 -> [w1018]
                        n413 = call "readbinary.vi"(7:w1018, "base path"=w1021, "file index"=w1022, "data column"=w1023) -> ("data"=w1026:ext[])  [unwired: 7 out]
                        n414 = Subtract(x=w1020, y=w1019) -> (x-y=w1027:i32)
                        n415 = Increment(x=w1027) -> (x+1=w1025:i32)
                        n416 = Array Subset(array=w1026, index=w1019, length=w1025) -> (w1024:ext[])
                        n417 = call "writebinary.vi"(7:w1018, "base path"=w1021, "file index"=w1022, "data column"=w1023, "data"=w1024) -> ()  [unwired: 7 out]
                      }
                    }
                  }
                }
              }
            }
          }
          frame #15 {
            n418 = And(x="?", y=w1031) -> (x .and. y?=w1029:bool)
            n419 = case shown="True" w1029 {
              tunnel: w1034 -> [_ w1038]
              tunnel: w1033 -> [_ w1037]
              tunnel: w1032 -> [_ w1036]
              tunnel: w1028 -> [_ w1035]
              frame False {
              }
              frame True {
                n420 = for {
                  tunnel: w1038 -> [w1041]
                  tunnel: w1036 -> [w1040]
                  tunnel: w1037 -> [_] mode=indexing
                  tunnel: w1035 -> [w1039]
                  i -> [w1042]
                  n421 = stacked-sequence {
                    seq-local: [w1046 _] -> [_ w1059]
                    tunnel: w1042 -> [w1053 w1061]
                    tunnel: w1041 -> [w1052 w1060]
                    tunnel: w1040 -> [_ w1062]
                    tunnel: w1039 -> [w1043 w1058]
                    frame #0 {
                      n422 = call "readbinary.vi"(7:w1043, "base path"=w1052, "file index"=w1053, "data column"="bcol") -> ("data"=w1050:ext[])  [unwired: 7 out]
                      n423 = case shown="True" "?" {
                        tunnel: w1050 -> [w1055 w1057]
                        tunnel: [w1055 w1056] -> w1049
                        frame False {
                        }
                        frame True {
                          n424 = Absolute Value(x=w1057) -> (abs(x)=w1056:ext[])
                        }
                      }
                      n425 = Greater Or Equal?(x=w1049, y="lower cutoff") -> (x >= y?=w1048:bool[])
                      n426 = Less Or Equal?(x=w1049, y="upper cutoff") -> (x <= y?=w1047:bool[])
                      n427 = And(x=w1048, y=w1047) -> (x .and. y?=w1046:bool[])
                    }
                    frame #1 {
                      n428 = for {
                        tunnel: w1062 -> [w1070] mode=indexing
                        tunnel: w1061 -> [w1069]
                        tunnel: w1060 -> [w1068]
                        tunnel: w1059 -> [w1067]
                        tunnel: w1058 -> [w1063]
                        n429 = call "readbinary.vi"(7:w1063, "base path"=w1068, "file index"=w1069, "data column"=w1070) -> ("data"=w1066:ext[])  [unwired: 7 out]
                        n430 = for {
                          tunnel: w1067 -> [w1074] mode=indexing
                          tunnel: w1066 -> [w1073] mode=indexing
                          shift-right: [w1071] -> w1064
                          shift-left: ext[] [] ("Array") -> [w1072]
                          n431 = case shown="True" w1074 {
                            tunnel: w1073 -> [_ w1078]
                            tunnel: w1072 -> [w1075 w1077]
                            tunnel: [w1075 w1076] -> w1071
                            frame False {
                            }
                            frame True {
                              n432 = Build Array (concatenate)(w1077, w1078) -> (w1076:ext[])
                            }
                          }
                        }
                        n433 = call "writebinary.vi"(7:w1063, "base path"=w1068, "file index"=w1069, "data column"=w1070, "data"=w1064) -> ()  [unwired: 7 out]
                      }
                    }
                  }
                }
              }
            }
          }
          frame #16 {
            w1083 = 0
            n434 = Equal?(x=w1103, y=3) -> (x = y?=w1098:bool)
            n435 = Equal?(x=w1099, y=1) -> (x = y?=w1097:bool)
            n436 = Array Size(array=w1100) -> (size(s)=w1091:i32)
            n437 = Greater Than 0?(x=w1091) -> (x > 0?=w1094:bool)
            n438 = And(x=w1098, y=w1097) -> (x .and. y?=w1093:bool)
            n439 = And(x=w1093, y=w1094) -> (x .and. y?=w1087:bool)
            n440 = In Range and Coerce(upper limit=w1091, x="file index", lower limit=0) -> (coerced(x)=w1089:i32, In Range?=w1088:bool)
            n441 = And(x=w1087, y=w1088) -> (x .and. y?=w1086:bool)
            n442 = case shown="False" "mode" {
              tunnel: w1102 -> [w1113 w1132]
              tunnel: w1101 -> [w1112 w1130]
              tunnel: w1100 -> [w1111 w1134]
              tunnel: w1096 -> [w1110 w1129]
              tunnel: w1089 -> [w1109 w1131]
              tunnel: w1086 -> [w1108 w1133]
              tunnel: [w1107 w1135] -> w1085
              frame False {
                n443 = case shown="True" w1108 {
                  tunnel: w1111 -> [_ w1122]
                  tunnel: w1113 -> [_ w1121]
                  tunnel: w1112 -> [_ w1120]
                  tunnel: [dbl[][] [] ("Array 9") w1119] -> w1105
                  tunnel: w1109 -> [_ w1118]
                  tunnel: w1110 -> [_ w1117]
                  tunnel: ["" w1116] -> w1107
                  frame False {
                  }
                  frame True {
                    n444 = Index Array(array=w1122, index=w1118) -> (element=w1116:string)
                    n445 = for {
                      tunnel: w1121 -> [w1127] mode=indexing
                      tunnel: w1118 -> [w1126]
                      tunnel: w1120 -> [w1125]
                      tunnel: [w1124] -> w1119 mode=indexing
                      tunnel: w1117 -> [w1123]
                      n446 = call "readbinary.vi"(7:w1123, "base path"=w1125, "file index"=w1126, "data column"=w1127) -> ("data"=w1124:ext[])  [unwired: 7 out]
                    }
                  }
                }
                n447 = Transpose 2D Array(2D array=w1105) -> (transposed array=w1106:ext[][])
                n448 = property class="Arr (strict)"("Val(Sgnl)"=w1106) -> ()  [unwired: 2 in, 2 out]
              }
              frame True {
                n449 = case shown="True" w1133 {
                  tunnel: w1134 -> [_ w1147]
                  tunnel: w1132 -> [_ _]
                  tunnel: w1130 -> [_ _]
                  tunnel: [dbl[][] [] ("Array 9") w1143] -> w1128
                  tunnel: w1131 -> [_ w1146]
                  tunnel: w1129 -> [_ _]
                  tunnel: ["" w1145] -> w1135
                  frame False {
                  }
                  frame True {
                    n450 = Index Array(array=w1147, index=w1146) -> (element=w1145:string)
                    n451 = Transpose 2D Array(2D array="?") -> (transposed array=w1143:T4)
                  }
                }
                n452 = for {
                  tunnel: w1132 -> [w1140] mode=indexing
                  tunnel: w1131 -> [w1139]
                  tunnel: w1130 -> [w1138]
                  tunnel: w1129 -> [w1137]
                  tunnel: w1128 -> [w1136] mode=indexing
                  n453 = call "writebinary.vi"(7:w1137, "base path"=w1138, "file index"=w1139, "data column"=w1140, "data"=w1136) -> ()  [unwired: 7 out]
                }
              }
            }
            "file" <- w1085
            n454 = property class="Arr (strict)"() -> ("Index Values"=w1081:u32[])  [unwired: 2 in, 2 out]
            n455 = Index Array(array=w1081, index=w1083) -> (element=w1084:u32)
            n456 = property class="Arr (strict)"("Number of Columns"=6) -> ()  [unwired: 2 in, 2 out]
            n457 = Build Array(w1084, w1083) -> (w1082:u32[])
            n458 = property class="Arr (strict)"("Index Values"=w1082) -> ()  [unwired: 2 in, 2 out]
          }
          frame #17 {
            w1149 = FALSE  # Set axes names
            n459 = Equal?(x=w1160, y=1) -> (x = y?=w1156:bool)
            n460 = Equal?(x=w1164, y=5) -> (x = y?=w1155:bool)
            n461 = Compound Arithmetic op=AND(w1156, w1155) -> (w1158:bool)
            n462 = case shown="True" w1158 {
              tunnel: w1152 -> [_ w1182]
              tunnel: w1162 -> [_ w1185]
              tunnel: w1161 -> [_ w1184]
              tunnel: [w1177 w1183] -> w1154
              tunnel: w1157 -> [_ w1181]
              frame False {
                w1179 = dbl[] [] ("Array 2")
                n463 = Bundle("Array 2"=w1179, "Array 2"=w1179) -> (w1178:cluster{"Array 2":dbl[], "Array 2":dbl[]})  [unwired: 1 out]
                n464 = Build Array(w1178) -> (w1177:cluster{"Array 2":dbl[], "Array 2":dbl[]}[])
              }
              frame True {
                n465 = for {
                  tunnel: w1182 -> [_] mode=indexing
                  tunnel: w1185 -> [w1194]
                  tunnel: w1184 -> [w1191]
                  tunnel: [w1187] -> w1183 mode=indexing
                  tunnel: w1181 -> [w1186]
                  i -> [w1190]
                  n466 = Index Array(array=w1194, index="y axis") -> (element=w1193:string)
                  n467 = Index Array(array=w1194, index="x axis") -> (element=w1192:string)
                  n468 = call "readbinary.vi"(7:w1186, "base path"=w1191, "file index"=w1190, "data column"=w1192) -> ("data"=w1189:ext[])  [unwired: 7 out]
                  n469 = call "readbinary.vi"(7:w1186, "base path"=w1191, "file index"=w1190, "data column"=w1193) -> ("data"=w1188:ext[])  [unwired: 7 out]
                  n470 = Bundle("data"=w1189, "data"=w1188) -> (w1187:cluster{"data":ext[], "data":ext[]})  [unwired: 1 out]
                }
                n471 = global write "status.vi" "String"("plotting imported data ") -> ()
              }
            }
            "?" <- w1154
            n472 = case shown="1" "label" {
              tunnel: w1152 -> [w1165 _ _]
              tunnel: [w1165 w1168 w1173] -> w1150
              frame 0, Default {
              }
              frame 1 {
                n473 = property on="angle theta (cos theta renorm.)" class="Arr (strict)"() -> ("Value"=w1169:ext[])  [unwired: 2 in, 2 out]
                n474 = Number To Fractional String(number=w1169, width (-)=10, precision (6)=3) -> (F-format string=w1168:string[])  [unwired: 1 out]
              }
              frame 2 {
                n475 = property on="variable (T)" class="Arr (strict)"() -> ("Value"=w1172:dbl[])  [unwired: 2 in, 2 out]
                n476 = Number To Fractional String(number=w1172, width (-)=10, precision (6)=3) -> (F-format string=w1173:string[])  [unwired: 1 out]
              }
            }
            n477 = control-ref of="?"() -> (w1151:refnum<vi>)
            n478 = while {
              stop <- w1175 stop-if-true
              n479 = Not(x="?") -> (.not. x?=w1175:bool)
              n480 = Wait (ms)(milliseconds to wait=1000) -> ()  [unwired: 1 out]
            }
            n481 = call "Neilsetplot.vi"("Set axes names"=w1149, "max # rows (-1:all)"=-1, "Plot names"=w1150, "XYGraph Refnum"=w1151) -> ()  [unwired: 6 in, 2 out]
          }
          frame #18 {
            n482 = case shown="True" "?" {
              tunnel: w1201 -> [_ w1216]
              tunnel: w1202 -> [_ w1215]
              tunnel: w1200 -> [_ w1213]
              tunnel: w1204 -> [_ w1208]
              tunnel: w1203 -> [_ w1212]
              tunnel: w1199 -> [_ w1211]
              tunnel: w1198 -> [w1206 w1210]
              tunnel: [w1206 w1209] -> w1197
              frame False {
              }
              frame True {
                n483 = for {
                  tunnel: w1216 -> [w1235] mode=indexing
                  tunnel: w1215 -> [w1233] mode=indexing
                  tunnel: "append name" -> [w1234]
                  tunnel: w1213 -> [w1229]
                  tunnel: w1208 -> [w1227]
                  tunnel: w1212 -> [w1224]
                  tunnel: w1211 -> [w1223]
                  shift-right: [w1221] -> w1209
                  shift-left: w1210 -> [w1219]
                  tunnel: w1208 -> [w1218]
                  i -> [w1228]
                  n484 = call "filecount.vi"("Path"=w1218) -> ("file count string"=w1217:string)  [unwired: 10 out]
                  n485 = Concatenate Strings("mega", w1217, w1235, w1234) -> (w1232:string)
                  n486 = Build Path(base path=w1233, name or relative path=w1232) -> (appended path=w1220:path)
                  n487 = Build Array (concatenate)(w1220, w1219) -> (w1221:path[])
                  n488 = Array Size(array=w1229) -> (size(s)=w1231:i32)
                  n489 = Decrement(x=w1231) -> (x-1=w1230:i32)
                  n490 = for {
                    N: w1230 -> [_]
                    tunnel: w1229 -> [w1252]
                    tunnel: w1228 -> [w1249]
                    tunnel: w1227 -> [w1248]
                    tunnel: [w1247] -> w1225 mode=indexing
                    tunnel: w1223 -> [w1246]
                    i -> [w1253]
                    n491 = Increment(x=w1253) -> (x+1=w1251:i32)
                    n492 = Index Array(array=w1252, index=w1251) -> (element=w1250:string)
                    n493 = call "readbinary.vi"(7:w1246, "base path"=w1248, "file index"=w1249, "data column"=w1250) -> ("data"=w1247:ext[])  [unwired: 7 out]
                  }
                  n494 = stacked-sequence {
                    tunnel: "time\tdB/dt\tBfield\tdata1\tdata2\n" -> [_ w1241 _]
                    tunnel: w1220 -> [w1236 w1240 w1244]
                    tunnel: w1225 -> [_ _ w1245]
                    tunnel: w1224 -> [_ _ w1243]
                    frame #0 {
